vi "Configure Slew Rate (Current).vi"(0 "VISA resource name":refnum<visa-resource-name>, 5 "Current Slew Rate (0 A per sec)":dbl format="%#.6f", 11 "error in (no error)":errorcluster) -> (4 "VISA resource name out":refnum<visa-resource-name>, 15 "error out":errorcluster)   [LabVIEW 2012, in "NH Research Regenerative Test Series.lvlib"]
doc: "Sets the slew rate for all programmed changes in the output current level of the module. This command programs both positive and negative going slew rates. Although any slew rate value may be entered, the module selects a slew rate that is closest to the programmed value. Slew rates less than the minimum value are set to minimum. Slew rates greater than the maximum value are set to maximum."
uses:
  <instrlib>/NH Research Regenerative Test Series/NH Research Regenerative Test Series.lvlib
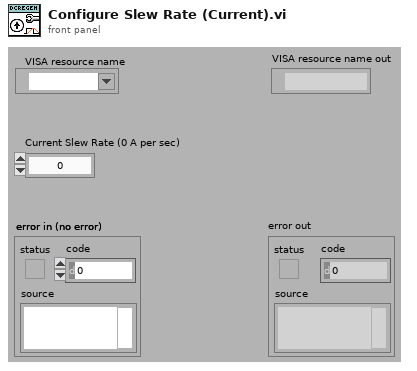
[diagram p1: front panel]
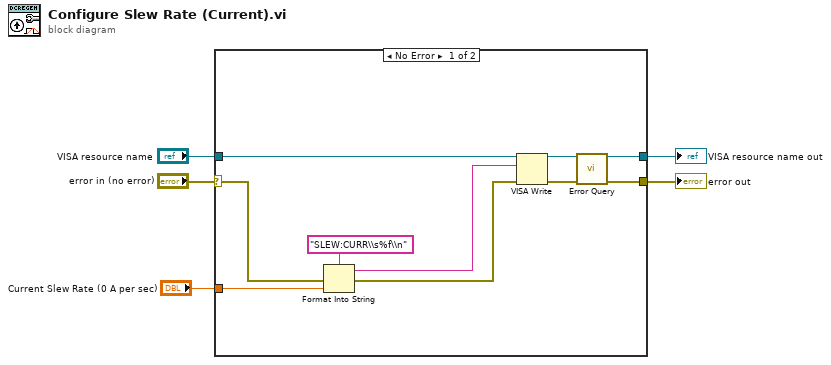
[diagram p0: block diagram]
diagram:
  n1 = case shown="No Error" "error in (no error)" {
    selector: "error in (no error)" -> [w9 w17]
    tunnel: "VISA resource name" -> [w15 w16]
    tunnel: [w14 w16] -> w4
    tunnel: [w13 w17] -> w3
    tunnel: "Current Slew Rate (0 A per sec)" -> [w10 _]
    frame No Error {
      n2 = Format Into String(format string="SLEW:CURR\\s%f\\n", error in=w9, w10) -> (resulting string=w7:string, error out=w8:errorcluster)  [unwired: 1 in]
      n3 = VISA Write(VISA resource name=w15, write buffer=w7, error in (no error)=w8) -> (VISA resource name out=w12:refnum<visa-resource-name>, error out=w11:errorcluster)  [unwired: 1 out]
      n4 = call <instrlib>:"Error Query.vi"("VISA resource name"=w12, "error in (no error)"=w11) -> ("VISA resource name out"=w14:refnum<visa-resource-name>, "error out"=w13:errorcluster)  [unwired: 10 in, 2 out]
    }
    frame Error {
    }
  }
  "error out" <- w3
  "VISA resource name out" <- w4
